vi "Signal Get Data.vi"(8 "error in (no error)":errorcluster, 11 "Signal DVR in":refnum<data-value>) -> (0 "error out":errorcluster, 2 "Data out":refnum<data-value>, 3 "Signal DVR out":refnum<data-value>)   [LabVIEW 2012, in "MDSplus.lvlib"]
uses:
  <vilib>/MDSplus/Library/MDSplus.lvlib
  <vilib>/MDSplus/Classes/Data_Class/Data.lvclass
  <vilib>/MDSplus/Classes/Data_Class/Compound_Class/Signal_Class/Signal.lvclass
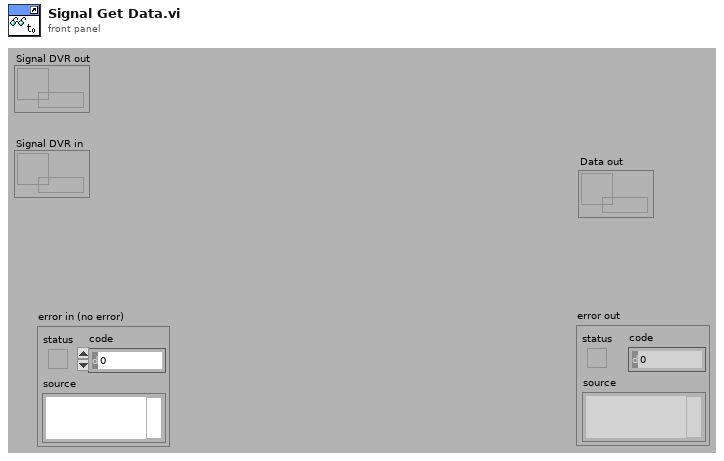
[diagram p1: front panel]
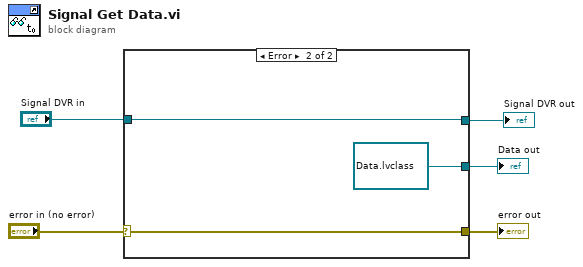
[diagram p0: block diagram]
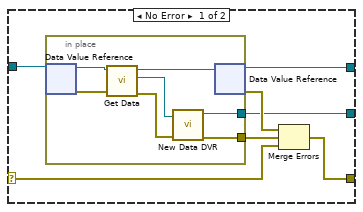
[diagram p2: hidden frame]
diagram:
  n1 = case shown="Error" "error in (no error)" {
    selector: "error in (no error)" -> [w12 w22]
    tunnel: [w9 w22] -> w5
    tunnel: [w10 w20] -> w1
    tunnel: [w7 refnum<data-value> refnum ("Data DVR")] -> w3
    tunnel: "Signal DVR in" -> [w6 w20]
    frame No Error {
      n2 = in-place {
        in-place-border: [w19] -> w7
        in-place-border: [w18] -> w8
        n3 = in-place-dvr #1(w6) -> (w17:refnum<class "Signal.lvclass">, w13:errorcluster)
        n4 = call-dynamic "Get Data.vi"("error in (no error)"=w13, "Signal in"=w17) -> ("error out"=w15:errorcluster, "Data out"=w14:refnum<class "Data.lvclass">, "Signal out"=w16:refnum<class "Signal.lvclass">)  [unwired: 7 in]
        n5 = call <vilib>:"New Data DVR.vi"("error in (no error)"=w15, "Data in"=w14) -> ("error out"=w18:errorcluster, "Data DVR out"=w19:refnum<data-value>)  [unwired: 8 in]
        n6 = in-place-dvr #1(w16) -> (w10:refnum<data-value>, w11:errorcluster)
      }
      n7 = Merge Errors(w11, w8, w12) -> (w9:errorcluster)
    }
    frame Error {
    }
  }
  "error out" <- w5
  "Data out" <- w3
  "Signal DVR out" <- w1
